vi "Pict_to_Graph.vi"(0 "Xo":i32=338, 1 "Width":i32, 2 "Yo":i32=168, 3 "Heigth":i32, 8 "X Scale.Range:Minimum":dbl, 9 "X Scale.Range:Maximum":dbl, 10 "Y Scale.Range:Minimum":dbl, 11 "Y Scale.Range:Maximum":dbl) -> (5 "CursorY":dbl format="%.2f", 7 "CursorX":dbl format="%.2f")   [LabVIEW 2011]
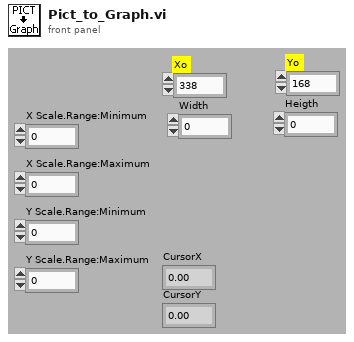
[diagram p1: front panel]
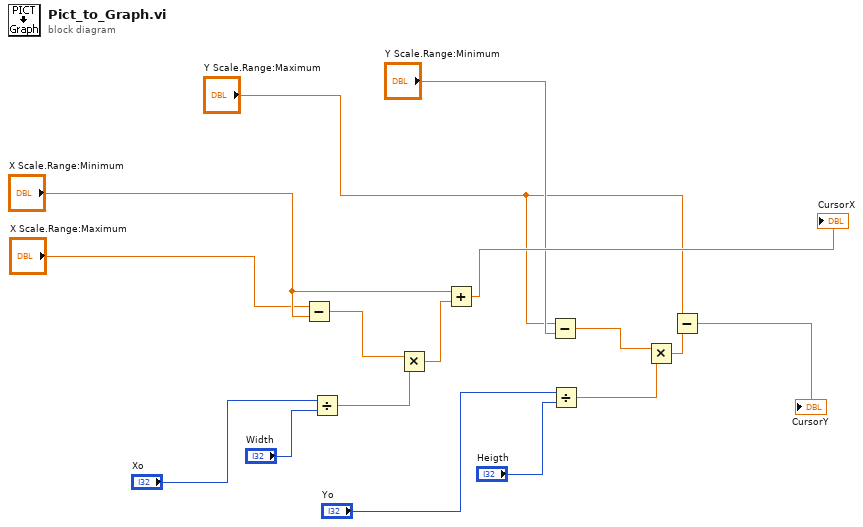
[diagram p0: block diagram]
diagram:
  n1 = Subtract(x="X Scale.Range:Maximum", y="X Scale.Range:Minimum") -> (x-y=w7:dbl)
  n2 = Divide(x="Xo", y="Width") -> (x/y=w15:dbl)
  n3 = Multiply(x=w7, y=w15) -> (x*y=w11:dbl)
  n4 = Add(x="X Scale.Range:Minimum", y=w11) -> (x+y=→"CursorX":dbl)
  n5 = Subtract(x="Y Scale.Range:Maximum", y="Y Scale.Range:Minimum") -> (x-y=w6:dbl)
  n6 = Divide(x="Yo", y="Heigth") -> (x/y=w14:dbl)
  n7 = Multiply(x=w6, y=w14) -> (x*y=w5:dbl)
  n8 = Subtract(x="Y Scale.Range:Maximum", y=w5) -> (x-y=→"CursorY":dbl)
